vi "Manual Climb.vi"(0 "Pull cable":bool, 1 "close arms":bool, 2 "Open arms + release cable":bool) -> ()   [LabVIEW 2012]
uses:
  Motors Values.vi
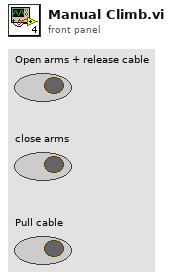
[diagram p1: front panel]
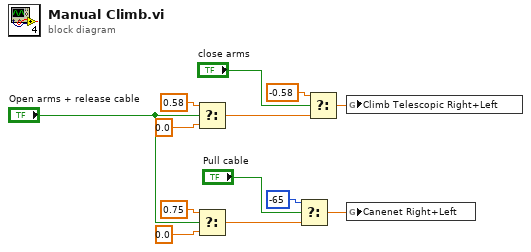
[diagram p0: block diagram]
diagram:
  n1 = Select(t=0.58, s="Open arms + release cable", f=0.0) -> (s? t:f=w9:dbl)
  n2 = Select(t=0.75, s="Open arms + release cable", f=0.0) -> (s? t:f=w5:dbl)
  n3 = Select(t=-65, s="Pull cable", f=w5) -> (s? t:f=w1:dbl)
  n4 = Select(t=-0.58, s="close arms", f=w9) -> (s? t:f=w2:dbl)
  n5 = global write "Motors Values.vi" "Climb Telescopic Right+Left"(w2) -> ()
  n6 = global write "Motors Values.vi" "Canenet Right+Left"(w1) -> ()
